vi "solar_qtimer Get.vi"(6 "Suppress Errors? (T)":bool=TRUE, 8 "error in (no error)":errorcluster, 10 "QTimer Name":string, 11 "QTimer Refnum in":T2) -> (0 "error out":errorcluster, 2 "Settings":T1={"QTimer"="", "Delay"=0, "Start"=FALSE, "EnQ_Type"=enum."IgnoreIfExists", "Messages"=[]}, 3 "QTimer Refnum out":T2)   [LabVIEW 2018]
doc: "This sets the start/stop of the QTimer by name."
uses:
  solar_qtimer_ctl Refnum.ctl
  solar_qtimer_ctl QTimer Settings.ctl
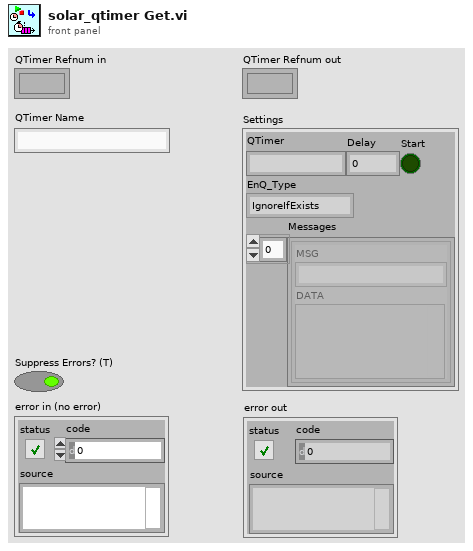
[diagram p1: front panel]
types:
  T1 = typedef "solar_qtimer_ctl QTimer Settings.ctl" = cluster{"QTimer":string, "Delay":i32, "Start":bool, "EnQ_Type":enum8{"Normal", "Priority", "IgnoreIfExists"}, "Messages":cluster{"MSG":string, "DATA":variant}[]}
  T2 = typedef "solar_qtimer_ctl Refnum.ctl" = refnum<k1>
  T3 = typedef "solar_qtimer_ctl SEQ.ctl" = cluster{"QTimers":T4[]}
  T4 = typedef "solar_qtimer_ctl QTimer.ctl" = cluster{"Settings":T1, "Queue":refnum<queue>, "QTimerQ":refnum<queue>, "VI Refnum":refnum<vi>}
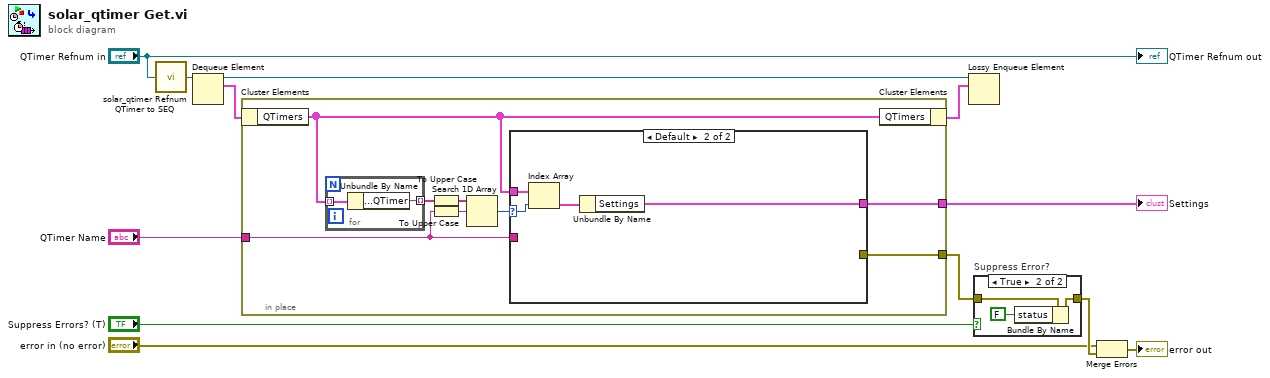
[diagram p0: block diagram]
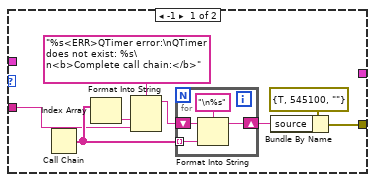
[diagram p2: hidden frame]
diagram:
  n1 = call "solar_qtimer Refnum QTimer to SEQ.vi"("QTimer Refnum"="QTimer Refnum in") -> ("QTimers SEQ"=w8:refnum<queue>)
  n2 = Dequeue Element(queue=w8) -> (queue out=w7:refnum<queue>, element=w6:T3)  [unwired: 2 in, 2 out]
  n3 = in-place {
    in-place-border: "QTimer Name" -> [w16]
    in-place-border: [w15] -> w3
    in-place-border: [w13] -> w1
    n4 = in-place-cluster #1(w6) -> ("QTimers"=w14:T4[])
    n5 = for {
      tunnel: w14 -> [w38] mode=indexing
      tunnel: [w37] -> w20 mode=indexing
      n6 = Unbundle By Name(w38) -> ("Settings.QTimer"=w37:string)
    }
    n7 = To Upper Case(1:w20) -> (0:w19:string[])
    n8 = To Upper Case(1:w16) -> (0:w18:string)
    n9 = Search 1D Array(1D array=w19, element=w18) -> (index of element=w17:i32)  [unwired: 1 in]
    n10 = case shown="Default" w17 {
      selector: w17 -> [_ w35]
      tunnel: w16 -> [w22 _]
      tunnel: [w21 _] -> w15
      tunnel: w14 -> [_ w36]
      tunnel: [_ w33] -> w13
      frame -1 {
        n11 = Call Chain() -> (call chain=w25:string[])
        n12 = Index Array(array=w25) -> (element=w27:string)  [unwired: 1 in]
        n13 = Format Into String(format string="%s<ERR>QTimer error:\nQTimer does not exist: %s\n<b>Complete call chain:</b>", w27, w22) -> (resulting string=w26:string)  [unwired: 2 in, 1 out]
        n14 = for {
          tunnel: w25 -> [w32] mode=indexing
          shift-right: [w31] -> w24
          shift-left: w26 -> [w30]
          n15 = Format Into String(format string="\n%s", initial string=w30, w32) -> (resulting string=w31:string)  [unwired: 1 in, 1 out]
        }
        n16 = Bundle By Name(cluster=errorcluster {"status"=TRUE, "code"=545100, "source"=""} ("error in (no error)"), "source"=w24) -> (w21:errorcluster)
      }
      frame Default {
        n17 = Index Array(array=w36, index=w35) -> (element=w34:T4)
        n18 = Unbundle By Name(w34) -> ("Settings"=w33:T1)
      }
    }
    n19 = in-place-cluster #1("QTimers"=w14) -> (w5:T3)
  }
  "Settings" <- w1
  n20 = Lossy Enqueue Element(queue=w7, element=w5) -> ()  [unwired: 1 in, 4 out]
  n21 = case "Suppress Error?" shown="True" "Suppress Errors? (T)" {
    tunnel: w3 -> [w39 w42]
    tunnel: [w39 w41] -> w11
    frame False {
    }
    frame True {
      n22 = Bundle By Name(cluster=w42, "status"=FALSE) -> (w41:errorcluster)
    }
  }
  n23 = Merge Errors("error in (no error)", w11) -> (→"error out":errorcluster)
  "QTimer Refnum out" <- "QTimer Refnum in"
